vi "get_component_type_name.vi"(8 "error in (no error)":errorcluster, 11 "GenericLightSource in":refnum<class "GenericLightSource.lvclass">) -> (0 "error out":errorcluster, 2 "component type":string="LightSource", 3 "GenericLightSource out":refnum<class "GenericLightSource.lvclass">)   [LabVIEW 2010, in "GenericLightSource.lvclass"]
uses:
  GenericLightSource.lvclass
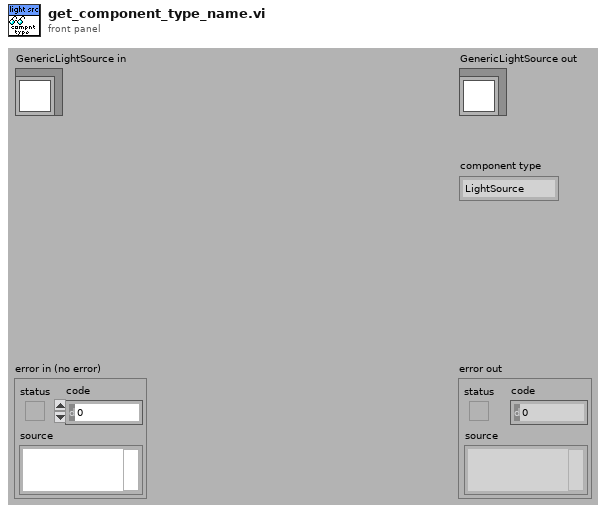
[diagram p1: front panel]
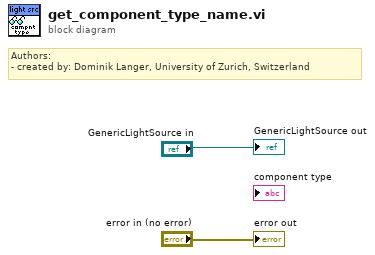
[diagram p0: block diagram]
diagram:
  # "Authors: \n- created by: Dominik Langer, University of Zurich, Switzerland"
  "error out" <- "error in (no error)"
  "GenericLightSource out" <- "GenericLightSource in"
